vi "Select OPC Channels.vi"(8 "error in (no error)":errorcluster, 11 "Node Ptr":u64 format="%.0x") -> (0 "error out":errorcluster)   [LabVIEW 2019, in "OPC UA Client Addon System Explorer.lvlib"]
uses:
  OPC UA Client Addon System Explorer.lvlib
  Types/Tag.SelectionMode.ctl
panel:
  in  "Tag":string
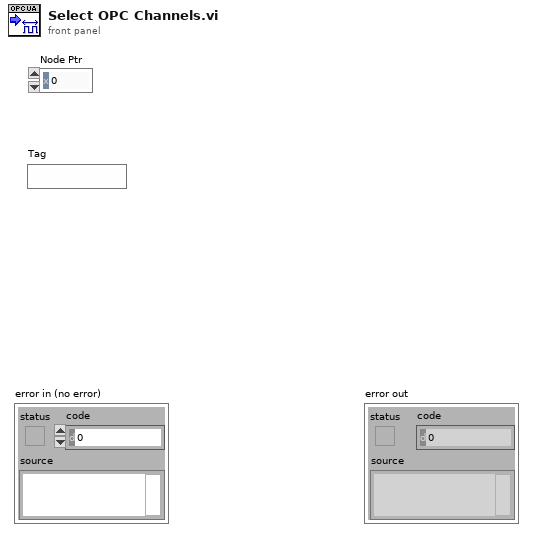
[diagram p1: front panel]
types:
  T1 = typedef "OPC UA Client Addon System Explorer.lvlib/Tag.SelectionMode.ctl" = enum8{"Live", "Offline"}
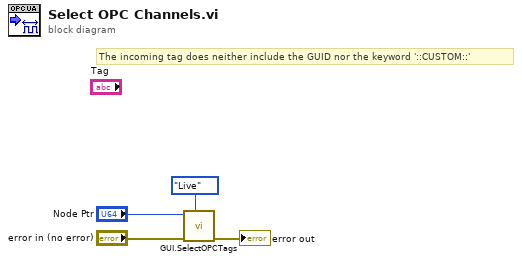
[diagram p0: block diagram]
diagram:
  # "The incoming tag does neither include the GUID nor the keyword '::CUSTOM::'"
  n1 = call "GUI.SelectOPCTags.vi"("Mode"=Tag.SelectionMode."Live", "error in"="error in (no error)", "Section Ptr"="Node Ptr") -> ("error out"=→"error out":errorcluster)  [unwired: 8 in]
